vi "Closest45rounding.vi"(1 "Gyro":dbl format="%#_13g") -> (0 "Closest Angle":dbl format="%#_13g")   [LabVIEW 2018]
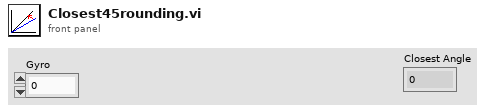
[diagram p1: front panel]
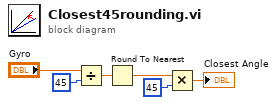
[diagram p0: block diagram]
diagram:
  n1 = Divide(x="Gyro", y=45) -> (x/y=w4:dbl)
  n2 = Round To Nearest(number=w4) -> (nearest integer value=w3:dbl)
  n3 = Multiply(x=w3, y=45) -> (x*y=→"Closest Angle":dbl)
